vi "testDrehmoment.vi"() -> ()   [LabVIEW 2014]
uses:
  <vilib>/CANopenLib/CANOPEN.llb/CANopen BaudRate.ctl
  <vilib>/CANopenLib/CANOPEN.llb/CANopen Interface Create.vi
  <vilib>/CANopenLib/CANOPEN.llb/CANopen SDO Create.vi
  <vilib>/CANopenLib/CANOPEN.llb/CANopen SDO Write [I8].vi
  <vilib>/CANopenLib/CANOPEN.llb/CANopen SDO Write [U16].vi
  <vilib>/CANopenLib/CANOPEN.llb/CANopen SDO Write [I16].vi
  <vilib>/CANopenLib/CANOPEN.llb/CANopen SDO Close.vi
  <vilib>/CANopenLib/CANOPEN.llb/CANopen Interface Close.vi
panel:
  in  "baud rate":T1 items=["1 Mbit/s"=0, "800 kbit/s"=1, "500 kbit/s"=2, "250 kbit/s"=3, "125 kbit/s"=4, "50 kbit/s"=6, "20 kbit/s"=7, "10 kbit/s"=8]
  in  "error in (no error)":errorcluster caption="Fehler (Eingang, kein Fehler)"
  out "error out":errorcluster
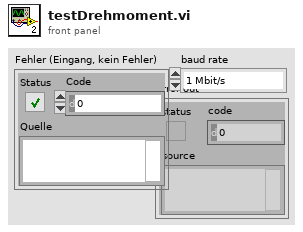
[diagram p1: front panel]
types:
  T1 = typedef "CANopen BaudRate.ctl" = u32
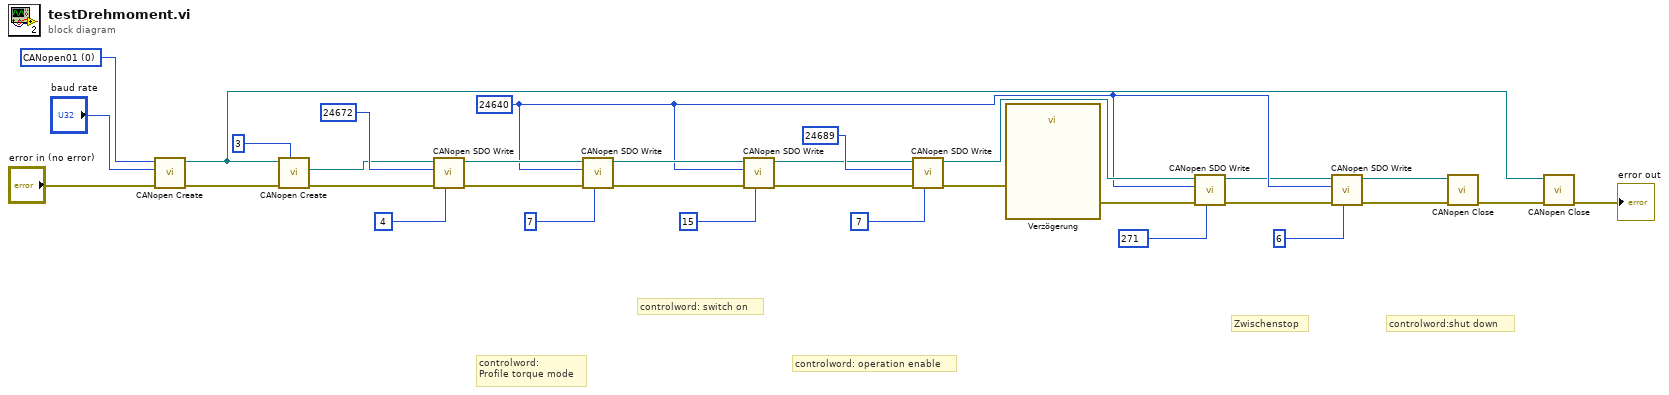
[diagram p0: block diagram]
diagram:
  w6 = u32 0 items=["CANopen01", "CANopen02", "CANopen03", "CANopen04", "CANopen05", "CANopen06", "CANopen07", "CANopen08", "CANopen09", "CANopen10", "CANopen11", "CANopen12", "CANopen13", "CANopen14", "CANopen15", "CANopen16", "CANopen17", "CANopen18", "CANopen19", "CANopen20", "CANopen21", "CANopen22", "CANopen23", "CANopen24", "CANopen25", "CANopen26", "CANopen27", "CANopen28", "CANopen29", "CANopen30", "CANopen31", "CANopen32"] ("interface name")
  w14 = u16 24640 ("object index")
  # "Zwischenstop"
  # "controlword:shut down"
  # "controlword: operation enable"
  # "controlword: switch on"
  # "controlword:\nProfile torque mode"
  n1 = call-poly <vilib>:"CANopen Create.vi"("error in (no error)"="error in (no error)", "baud rate"="baud rate", "interface name"=w6) -> ("error out"=w4:errorcluster, "interface object out"=w1:refnum<k20>)  [unwired: 7 in]
  n2 = call-poly <vilib>:"CANopen Create.vi"("node-ID"=u8 3, "error in (no error)"=w4, "interface object in"=w1) -> ("error out"=w28:errorcluster, "SDO object out"=w29:refnum<k20>)  [unwired: 6 in, 1 out]
  n3 = call-poly <vilib>:"CANopen SDO Write.vi"("I8 data"=i8 4, "error in (no error)"=w28, "object index"=u16 24672, "SDO object in"=w29) -> ("error out"=w24:errorcluster, "SDO object out"=w25:refnum<k20>)  [unwired: 5 in, 1 out]
  n4 = call-poly <vilib>:"CANopen SDO Write.vi"("U16 data"=u16 7, "error in (no error)"=w24, "object index"=w14, "SDO object in"=w25) -> ("error out"=w22:errorcluster, "SDO object out"=w23:refnum<k20>)  [unwired: 5 in, 1 out]
  n5 = call-poly <vilib>:"CANopen SDO Write.vi"("U16 data"=u16 15, "error in (no error)"=w22, "object index"=w14, "SDO object in"=w23) -> ("error out"=w18:errorcluster, "SDO object out"=w19:refnum<k20>)  [unwired: 5 in, 1 out]
  n6 = call-poly <vilib>:"CANopen SDO Write.vi"("I16 data"=i16 7, "error in (no error)"=w18, "object index"=u16 24689, "SDO object in"=w19) -> ("error out"=w17:errorcluster, "SDO object out"=w15:refnum<k20>)  [unwired: 5 in, 1 out]
  n7 = call "Verzögerung"("error in (no error)"=w17) -> ("error out"=w10:errorcluster)  [unwired: 10 in]
  n8 = call-poly <vilib>:"CANopen SDO Write.vi"("U16 data"=u16 271, "error in (no error)"=w10, "object index"=w14, "SDO object in"=w15) -> ("error out"=w12:errorcluster, "SDO object out"=w13:refnum<k20>)  [unwired: 5 in, 1 out]
  n9 = call-poly <vilib>:"CANopen SDO Write.vi"("U16 data"=u16 6, "error in (no error)"=w12, "object index"=w14, "SDO object in"=w13) -> ("error out"=w9:errorcluster, "SDO object out"=w8:refnum<k20>)  [unwired: 5 in, 1 out]
  n10 = call-poly <vilib>:"CANopen Close.vi"("error in (no error)"=w9, "SDO object in"=w8) -> ("error out"=w3:errorcluster)  [unwired: 9 in]
  n11 = call-poly <vilib>:"CANopen Close.vi"("error in (no error)"=w3, "interface object in"=w1) -> ("error out"=→"error out":errorcluster)  [unwired: 9 in]
